vi "File Append.vi"(2 "file path":path, 3 "String":string="1") -> ()   [LabVIEW 2016]
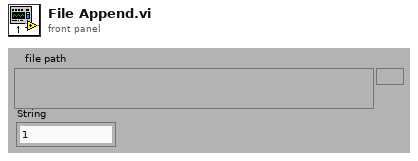
[diagram p1: front panel]
types:
  T1 = enum16{"open", "open or create", "create or replace", "create", "open (read only)"}
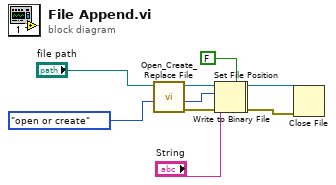
[diagram p0: block diagram]
diagram:
  n1 = call <vilib>:"Open_Create_Replace File.vi"("function (open:0)"=T1."open or create", "file path"="file path") -> ("error out"=w9:errorcluster, "file size (bytes)"=w7:i32, "refnum"=w8:refnum<file>)  [unwired: 6 in, 1 out]
  n2 = Set File Position(offset (in bytes) (0)=w7, refnum=w8, error in=w9) -> (refnum out=w4:refnum<file>, error out=w3:errorcluster)  [unwired: 1 in]
  n3 = Write to Binary File(file (use dialog)=w4, data="String", error in=w3, 5:FALSE ("prepend array or string size? (T)")) -> (refnum out=w5:refnum<file>, error out=w6:errorcluster)  [unwired: 2 in, 1 out]
  n4 = Close File(refnum=w5, error in=w6) -> ()  [unwired: 2 out]
